vi "Write Resource.vi"(8 "error in":errorcluster, 10 "Resource":refnum<visa-resource-name>, 11 "PIOD in":refnum<class "PIOD.lvclass">) -> (0 "error out":errorcluster, 3 "PIOD out":refnum<class "PIOD.lvclass">)   [LabVIEW 2018, in "PIOD.lvlib" / "PIOD.lvclass"]
uses:
  PIOD.lvclass
  C:/Users/Ron.Dexter.LUMINARTECH/Desktop/builds/PLC.lvlibp/PLC.lvclass
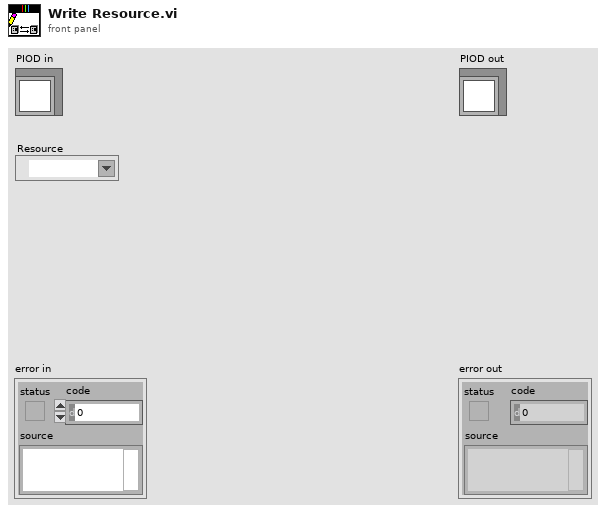
[diagram p1: front panel]
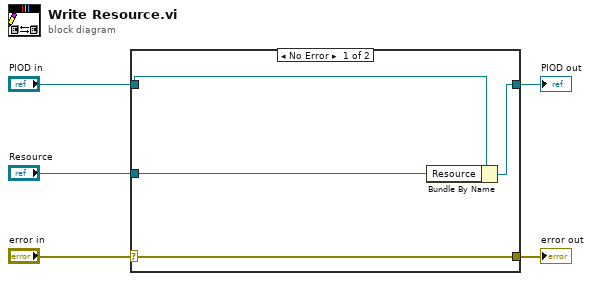
[diagram p0: block diagram]
diagram:
  n1 = case shown="No Error" "error in" {
    selector: "error in" -> [w9 w10]
    tunnel: [w9 w10] -> w4
    tunnel: [w7 w11] -> w2
    tunnel: "PIOD in" -> [w8 w11]
    tunnel: "Resource" -> [w6 _]
    frame No Error {
      n2 = Bundle By Name(cluster=w8, "Resource"=w6) -> (w7:refnum<class "PIOD.lvclass">)
    }
    frame Error {
    }
  }
  "error out" <- w4
  "PIOD out" <- w2
